vi "Fake Client Id Generator.vi"(8 "error in":errorcluster, 11 "action":T1) -> (0 "error out":errorcluster, 3 "client id":u64)   [LabVIEW 2020, in "MeasurementServerTests.lvlib" / "Discovery Tests.lvlib"]
uses:
  Discovery Tests.lvlib
  Fake Client Id Generator Action.ctl
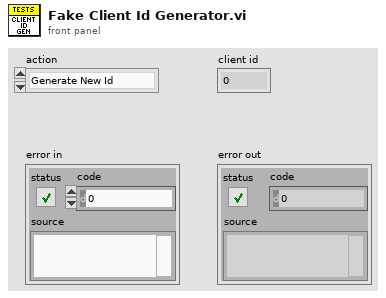
[diagram p1: front panel]
types:
  T1 = typedef "MeasurementServerTests.lvlib/Discovery Tests.lvlib/Fake Client Id Generator Action.ctl" = enum16{"Generate New Id", "Reset", "Error on Next Call"}
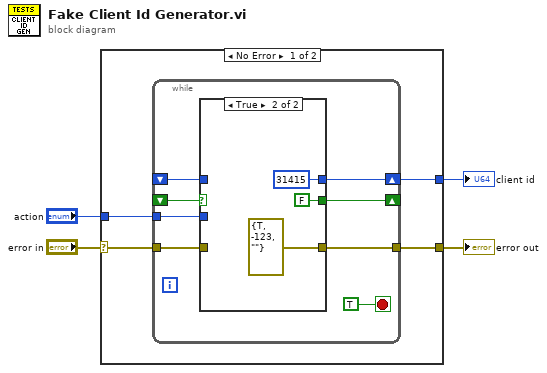
[diagram p0: block diagram]
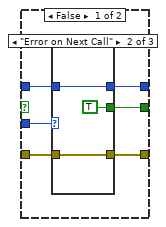
[diagram p2: hidden frame]
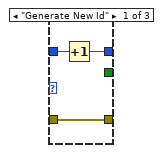
[diagram p3: hidden frame]
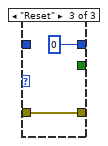
[diagram p4: hidden frame]
diagram:
  n1 = case shown="No Error" "error in" {
    selector: "error in" -> [w6 w34]
    tunnel: [w5 w34] -> w3
    tunnel: "action" -> [w8 _]
    tunnel: [w7 _] -> w2
    frame No Error {
      n2 = while {
        shift-right: [w15] -> w7
        shift-left: _ -> [w13]
        tunnel: w8 -> [w14]
        tunnel: w6 -> [w12]
        tunnel: [w11] -> w5
        shift-right: [w10] -> _
        shift-left: _ -> [w9]
        stop <- TRUE stop-if-true
        n3 = case shown="True" w9 {
          tunnel: [w22 u64 31415] -> w15
          tunnel: w14 -> [w21 _]
          tunnel: w13 -> [w20 _]
          tunnel: w12 -> [w19 _]
          tunnel: [w18 errorcluster {"status"=TRUE, "code"=-123, "source"=""} ("error IO")] -> w11
          tunnel: [w17 FALSE] -> w10
          frame False {
            n4 = case shown="\"Error on Next Call\"" w21 {
              tunnel: [w24 w28 u64 0] -> w22
              tunnel: w20 -> [w25 w28 _]
              tunnel: w19 -> [w23 w27 w29]
              tunnel: [w23 w27 w29] -> w18
              tunnel: [_ TRUE _] -> w17
              frame "Generate New Id" {
                n5 = Increment(x=w25) -> (x+1=w24:u64)
              }
              frame "Error on Next Call" {
              }
              frame "Reset" {
              }
            }
          }
          frame True {
          }
        }
      }
    }
    frame Error {
    }
  }
  "error out" <- w3
  "client id" <- w2
